vi "Flush Data to TDMS File.vi"(8 "error in (no error)":errorcluster, 10 "Data Queue":refnum<queue>, 11 "Logging Configuration":T3) -> (0 "error out":errorcluster, 3 "remaining elements":T1[](array[typedef]))   [LabVIEW 2022 SP3, in "Logging.lvlib"]
doc: "Flush the data queue of any pending data and write it to the log file. Close the TDMS file reference."
uses:
  Logging.lvlib
  QueuedLoggedData.ctl
  FFT-Data.ctl
  Logging Configuration.ctl
  support/TDMS-Refs.ctl
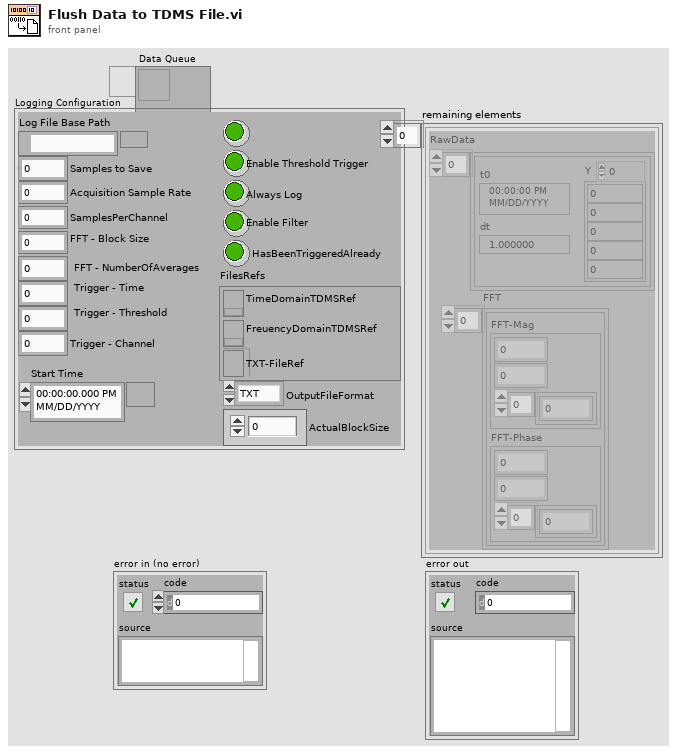
[diagram p1: front panel]
types:
  T1 = typedef "QueuedLoggedData.ctl" = cluster{"RawData":waveform(dbl)[], "FFT ":T2[]}
  T2 = typedef "FFT-Data.ctl" = cluster{"FFT-Mag":cluster{"t0":dbl, "dt":dbl, "Y":dbl[]}, "FFT-Phase":cluster{"t0":dbl, "dt":dbl, "Y":dbl[]}}
  T3 = typedef "Logging.lvlib/Logging Configuration.ctl" = cluster{"Log File Base Path":path, "Samples to Save":u32, "Acquisition Sample Rate":dbl, "SamplesPerChannel":u32, "FFT - Block Size":u32, "FFT - NumberOfAverages":i32, "Trigger - Time":i32, "Trigger - Threshold":dbl, "Trigger - Channel":u32, "Enable Time Trigger":bool, "Enable Threshold Trigger":bool, "Always Log":bool, "Enable Filter":bool, "FilesRefs":T4, "OutputFileFormat":enum16{"TXT", "TDMS"}, "ActualBlockSize":i32, "HasBeenTriggeredAlready":bool, "Start Time":timestamp}
  T4 = typedef "TDMS-Refs.ctl" = cluster{"TimeDomainTDMSRef":refnum<k34>, "FreuencyDomainTDMSRef":refnum<k34>, "TXT-FileRef":refnum<file>}
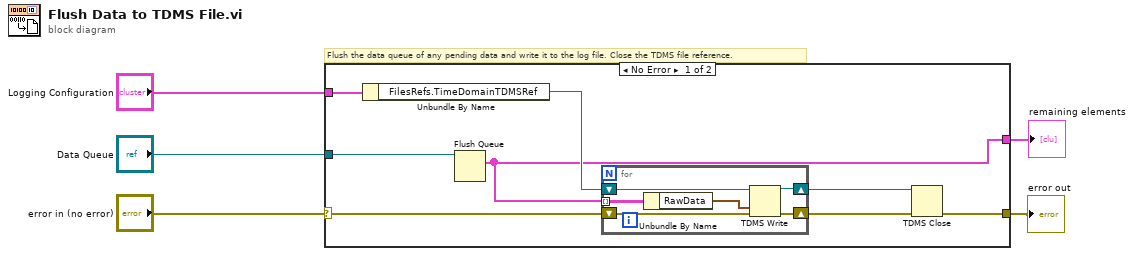
[diagram p0: block diagram]
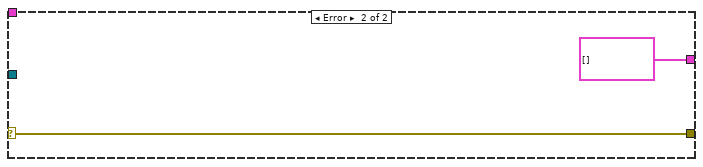
[diagram p2: hidden frame]
diagram:
  # "Flush the data queue of any pending data and write it to the log file. Close the TDMS file reference."
  n1 = case shown="No Error" "error in (no error)" {
    selector: "error in (no error)" -> [w8 w21]
    tunnel: "Data Queue" -> [w10 _]
    tunnel: "Logging Configuration" -> [w9 _]
    tunnel: [w7 w21] -> w3
    tunnel: [w6 T1[] [] ("remaining elements")] -> w1
    frame No Error {
      n2 = Unbundle By Name(w9) -> ("FilesRefs.TimeDomainTDMSRef"=w11:refnum<k34>)
      n3 = Flush Queue(queue=w10) -> (remaining elements=w6:T1[])  [unwired: 1 in, 2 out]
      n4 = for {
        shift-right: [w16] -> w12
        shift-left: w11 -> [w17]
        shift-right: [w18] -> w13
        shift-left: w8 -> [w19]
        tunnel: w6 -> [w15] mode=indexing
        n5 = Unbundle By Name(w15) -> ("RawData"=w14:waveform(dbl)[])
        n6 = TDMS Write(0:w17, 9:w14, 11:w19) -> (4:w16:refnum<k34>, 15:w18:errorcluster)  [unwired: 3 in, 2 out]
      }
      n7 = TDMS Close(8:w13, 11:w12) -> (0:w7:errorcluster)  [unwired: 1 out]
    }
    frame Error {
    }
  }
  "error out" <- w3
  "remaining elements" <- w1
